vi "GetAreaScanAxesRanges.vi"(0 "System no.":i32=1 min=1 max=4 step=1, 5 "error in":errorcluster) -> (14 "Scan Ranges":T1(array[cluster]), 19 "error out":errorcluster)   [LabVIEW 2020]
doc: "This VI reads all area scan routines from controller and calculates the scan ranges."
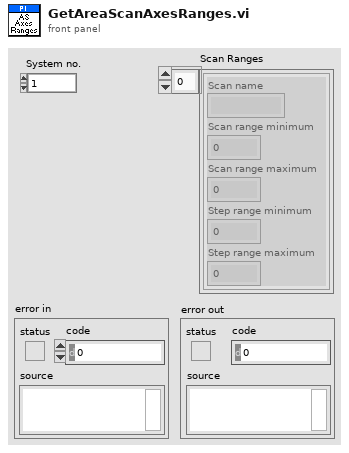
[diagram p1: front panel]
types:
  T1 = cluster{"Scan name":string, "Scan range minimum":dbl, "Scan range maximum":dbl, "Step range minimum":dbl, "Step range maximum":dbl}[]
  T2 = cluster{"Scan name":string, "Scan range minimum":dbl, "Scan range maximum":dbl, "Step range minimum":dbl, "Step range maximum":dbl}
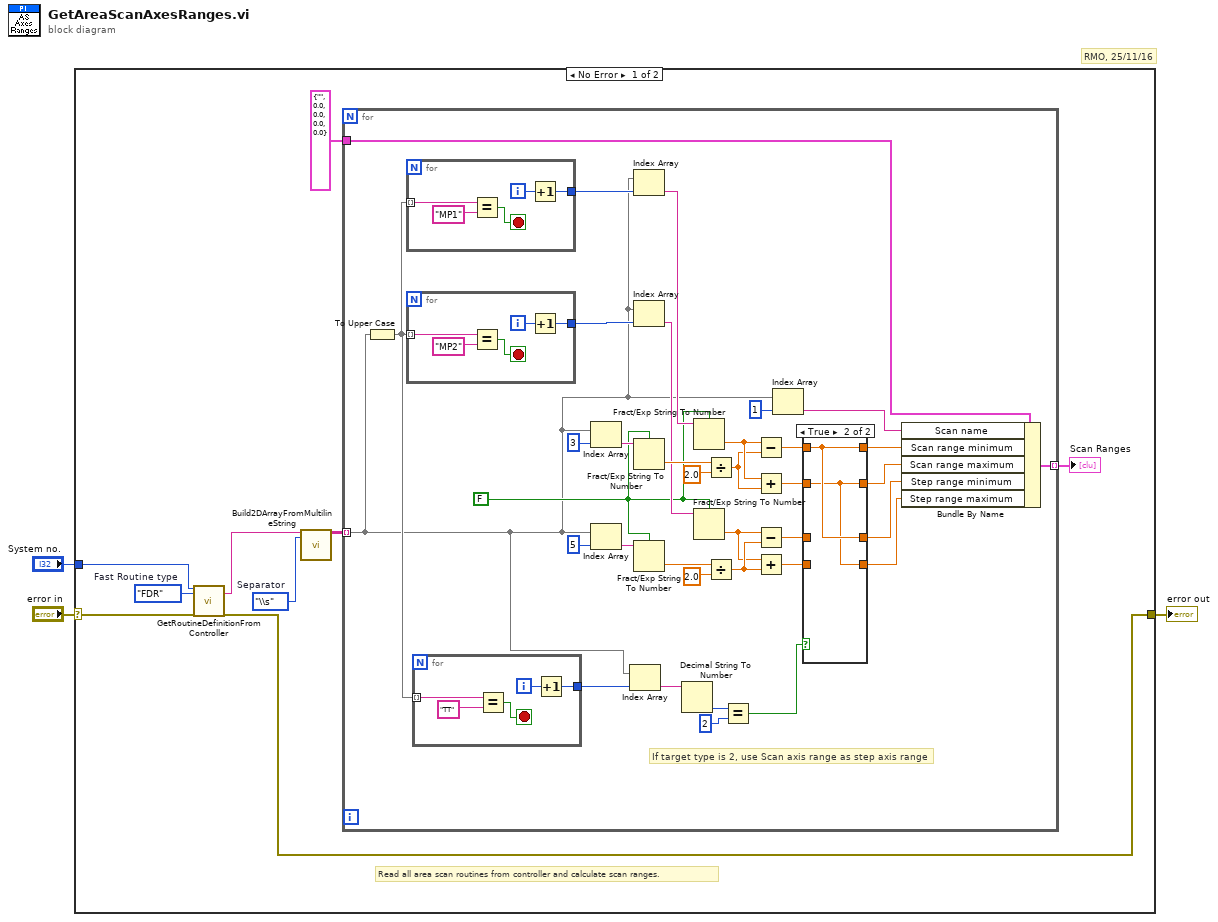
[diagram p0: block diagram]
diagram:
  # "RMO, 25/11/16"
  n1 = case shown="No Error" "error in" {
    selector: "error in" -> [w11 w70]
    tunnel: [w4 w70] -> w3
    tunnel: "System no." -> [w9 _]
    frame No Error {
      w8 = enum16{"FDG", "FDR"}."FDR"  # Fast Routine type
      w12 = enum16{"\\s", "\\t"}."\\s"  # Separator
      # "Read all area scan routines from controller and calculate scan ranges."
      n2 = call "GetRoutineDefinitionFromController.vi"("System no."=w9, "Fast Routine type"=w8, "error in"=w11) -> ("Routine Definitons"=w5:string, "error out"=w4:errorcluster)  [unwired: 15 out]
      n3 = call "Build2DArrayFromMultilineString.vi"("String"=w5, "Separator"=w12) -> ("2D Array out"=w10:string[][])  [unwired: 17 out]
      n4 = for {
        tunnel: w10 -> [w25] mode=indexing
        tunnel: T2 {"Scan name"="", "Scan range minimum"=0.0, "Scan range maximum"=0.0, "Step range minimum"=0.0, "Step range maximum"=0.0} ("Scan range") -> [w30]
        tunnel: [w28] -> w6 mode=indexing
        w31 = FALSE
        # "If target type is 2, use Scan axis range as step axis range"
        n5 = To Upper Case(1:w25) -> (0:w27:string[])
        n6 = for {
          tunnel: w27 -> [w69] mode=indexing
          tunnel: [w65] -> w45
          i -> [w66]
          stop <- w67 stop-if-true
          n7 = Equal?(x=w69, y="MP1") -> (x = y?=w67:bool)
          n8 = Increment(x=w66) -> (x+1=w65:i32)
        }
        n9 = for {
          tunnel: w27 -> [w64] mode=indexing
          tunnel: [w60] -> w44
          i -> [w61]
          stop <- w62 stop-if-true
          n10 = Equal?(x=w64, y="MP2") -> (x = y?=w62:bool)
          n11 = Increment(x=w61) -> (x+1=w60:i32)
        }
        n12 = for {
          tunnel: w27 -> [w59] mode=indexing
          tunnel: [w55] -> w26
          i -> [w56]
          stop <- w57 stop-if-true
          n13 = Equal?(x=w59, y="TT") -> (x = y?=w57:bool)
          n14 = Increment(x=w56) -> (x+1=w55:i32)
        }
        n15 = Index Array(array=w25, index=3 ("length")) -> (element=w43:string)
        n16 = Index Array(array=w25, index=5 ("length")) -> (element=w33:string)
        n17 = Index Array(array=w25, index=w26) -> (element=w24:string)
        n18 = Index Array(array=w25, index=w45) -> (element=w42:string)
        n19 = Index Array(array=w25, index=w44) -> (element=w32:string)
        n20 = Fract/Exp String To Number(use system decimal point (T)=w31, string=w43) -> (number=w41:dbl)  [unwired: 3 out]
        n21 = Fract/Exp String To Number(use system decimal point (T)=w31, string=w33) -> (number=w34:dbl)  [unwired: 3 out]
        n22 = Decimal String To Number(string=w24) -> (number=w23:i32)  [unwired: 3 out]
        n23 = Fract/Exp String To Number(use system decimal point (T)=w31, string=w42) -> (number=w39:dbl)  [unwired: 3 out]
        n24 = Fract/Exp String To Number(use system decimal point (T)=w31, string=w32) -> (number=w36:dbl)  [unwired: 3 out]
        n25 = Divide(x=w41, y=2.0) -> (x/y=w38:dbl)
        n26 = Divide(x=w34, y=2.0) -> (x/y=w37:dbl)
        n27 = Equal?(x=w23, y=2) -> (x = y?=w21:bool)
        n28 = Subtract(x=w39, y=w38) -> (x-y=w20:dbl)
        n29 = Add(x=w39, y=w38) -> (x+y=w18:dbl)
        n30 = Subtract(x=w36, y=w37) -> (x-y=w16:dbl)
        n31 = Add(x=w36, y=w37) -> (x+y=w14:dbl)
        n32 = Index Array(array=w25, index=1) -> (element=w29:string)
        n33 = case shown="True" w21 {
          tunnel: w20 -> [w52 w54]
          tunnel: [w52 w54] -> w19
          tunnel: w18 -> [w51 w53]
          tunnel: [w51 w53] -> w17
          tunnel: w16 -> [w50 _]
          tunnel: [w50 w54] -> w15
          tunnel: w14 -> [w49 _]
          tunnel: [w49 w53] -> w13
          frame False {
          }
          frame True {
          }
        }
        n34 = Bundle By Name(cluster=w30, "Scan name"=w29, "Scan range minimum"=w19, "Scan range maximum"=w17, "Step range minimum"=w15, "Step range maximum"=w13) -> (w28:T2)
      }
      "Scan Ranges" <- w6
    }
    frame Error {
    }
  }
  "error out" <- w3
